vi "Insert Case Structure.vi"(8 "error in (no error)":errorcluster, 10 "Insert Case Structure":T1, 11 "Test Executive Builder Model in":refnum<class "Test Executive Builder Model.lvclass">) -> (0 "error out":errorcluster, 3 "Test Executive Builder Model out":refnum<class "Test Executive Builder Model.lvclass">, 5 "Unique ID out":string)   [LabVIEW 2019, in "Test Executive Builder Model.lvclass"]
uses:
  <vilib>/gpm_packages/@cs/Test-executive-builder/Source/Test Executive Builder Model/Test Executive Builder Model/Test Executive Builder Model.lvclass
  C:/Program Files/National Instruments/LabVIEW 2019/vi.lib/ActorFramework/Actor/Actor.lvclass
  <vilib>/gpm_packages/@cs/Test-executive-builder/Source/Application Dependencies/Insert Case Structure.ctl
  <vilib>/gpm_packages/@cs/run-time-assertions/Source/Assert/Assert.lvclass
  <vilib>/gpm_packages/@cs/Test-executive-builder/Source/Test Executive Builder Model/Test Executive Builder Model/Test Executive Builder Model.lvclass/Test Executive Builder Model.ctl
  <vilib>/ActorFramework/Actor/Actor.lvclass/Actor.ctl
  <vilib>/ActorFramework/Message Enqueuer/Message Enqueuer.lvclass/Message Enqueuer.ctl
  <vilib>/ActorFramework/Message Enqueuer/Init from Existing Queue.vi
  <vilib>/ActorFramework/Message Enqueuer/Enqueue.vi
  <vilib>/gpm_packages/@cs/Test-executive-builder/Source/Test Executive Builder Model/Test Executive Builder Model Messages/Redraw Tree Msg/Redraw Tree Msg.lvclass
  C:/Program Files/National Instruments/LabVIEW 2019/vi.lib/ActorFramework/Message/Message.lvclass
  <vilib>/ActorFramework/Message Priority Queue/Priority Enqueue.vi
  <vilib>/ActorFramework/Message Enqueuer/Message Enqueuer.lvclass
  <vilib>/gpm_packages/@cs/test-executive/Source/Test Executive/TestExecutive Ref/TestExecutive Ref.lvclass
  <vilib>/ActorFramework/Actor/Actor.lvclass
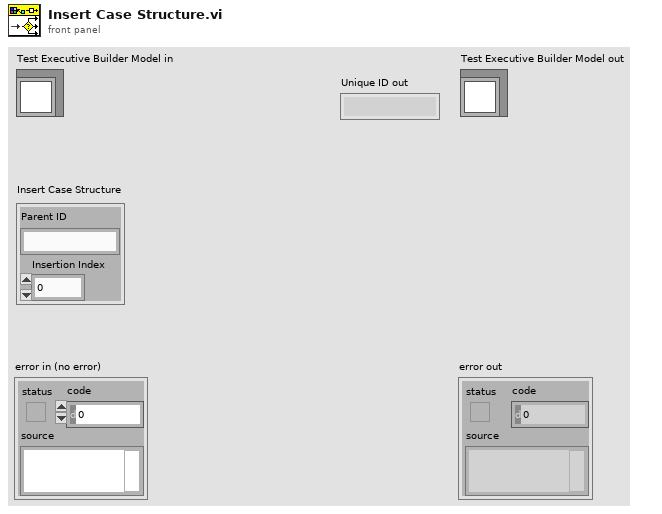
[diagram p1: front panel]
types:
  T1 = typedef "Insert Case Structure.ctl" = cluster{"Parent ID":string, "Insertion Index":i32}
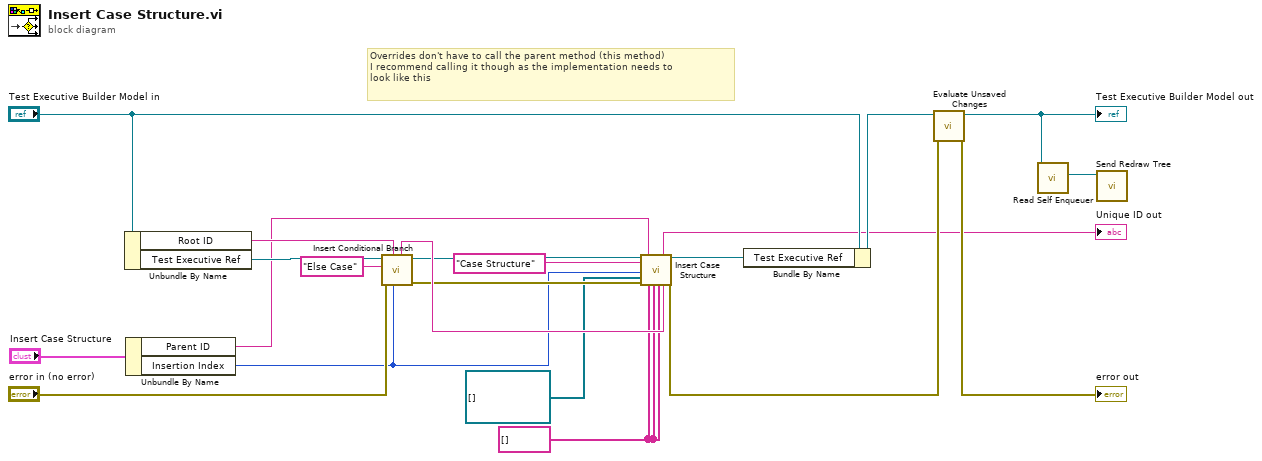
[diagram p0: block diagram]
diagram:
  w2 = string[] [] ("X Variables")
  # "Overrides don't have to call the parent method (this method)\nI recommend calling it though as the implementation needs to\nlook like this"
  n1 = Unbundle By Name("Test Executive Builder Model in") -> ("Root ID"=w19:string, "Test Executive Ref"=w21:refnum<data-value>)
  n2 = Unbundle By Name("Insert Case Structure") -> ("Parent ID"=w10:string, "Insertion Index"=w4:i32)
  n3 = call <vilib>:"Insert Conditional Branch.vi"("Insertion Index"=w4, "Parent ID"=w19, "error in (no error)"="error in (no error)", "Name"="Else Case", "Test Executive Ref"=w21) -> ("error out"=w5:errorcluster, "Test Executive Ref out"=w6:refnum<data-value>, "Unique ID out"=w7:string)  [unwired: 3 in, 1 out]
  n4 = call <vilib>:"Insert Case Structure.vi"("Test Executive Ref"=w6, "Name"="Case Structure", "Insertion Index"=w4, "Assertions"=refnum<class "Assert.lvclass">[] [], "error in (no error)"=w5, "Parent ID"=w10, "X Variables"=w2, "Y Variables"=w2, "Conditional Branches"=w2, "\"Else\" Conditional Branch"=w7) -> ("Unique ID out"=→"Unique ID out":string, "Test Executive Ref out"=w11:refnum<data-value>, "error out"=w12:errorcluster)  [unwired: 6 in, 1 out]
  n5 = Bundle By Name(cluster="Test Executive Builder Model in", "Test Executive Ref"=w11) -> (w15:refnum<class "Test Executive Builder Model.lvclass">)
  n6 = call-dynamic "Evaluate Unsaved Changes.vi"("error in (no error)"=w12, "Test Executive Builder Model in"=w15) -> ("error out"=→"error out":errorcluster, "Test Executive Builder Model out"=w14:refnum<class "Test Executive Builder Model.lvclass">)  [unwired: 8 in]
  "Test Executive Builder Model out" <- w14
  n7 = call <vilib>:"Read Self Enqueuer.vi"("Actor"=w14) -> ("Self Enqueuer"=w16:refnum<class "Message Enqueuer.lvclass">)  [unwired: 10 in]
  n8 = call <vilib>:"Send Redraw Tree.vi"("Message Enqueuer"=w16) -> ()  [unwired: 9 in, 2 out]
